vi "写入A1外设配置.vi"(8 "error in (no error)":errorcluster, 10 "外设配置":T1 {"总氮x公式0" items=["0", "1"]; "光谱仪类型" items=["1型", "2型", "3型", "2型氙灯联控"]; "泵阀量" items=["9通"=9, "10通"=10, "12通"=12]; "泵类型" items=["1型", "2型", "sy04型+旋转阀"]}, 11 "MB session in":refnum<class "MB_Master.lvclass">) -> (0 "error out":errorcluster, 3 "MB session out":refnum<class "MB_Master.lvclass">)   [LabVIEW 2016, in "斯坦道总磷总氮.lvlib"]
uses:
  <vilib>/Plasmionique/MB Master/MB_Master/MB_Master.lvclass
  <vilib>/Plasmionique/MB Master/MB_Master_Serial/MB_Master_Serial.lvclass
  C:/Program Files (x86)/National Instruments/LabVIEW 2016/vi.lib/Plasmionique/MB Master/MB_Master/MB_Master.lvclass
  <vilib>/Plasmionique/MB Master/MB Master.lvlib
  <vilib>/Utility/VariantDataType/VariantType.lvlib
panel:
  in  "U32":u32
  in  "SGL":sgl
  in  "U16":u16
  in  "U8":u8
  in  "VISA Resource":refnum<visa-resource-name>
  in  "引用选择":enum16{"MB引用", "自建引用"}(ring)
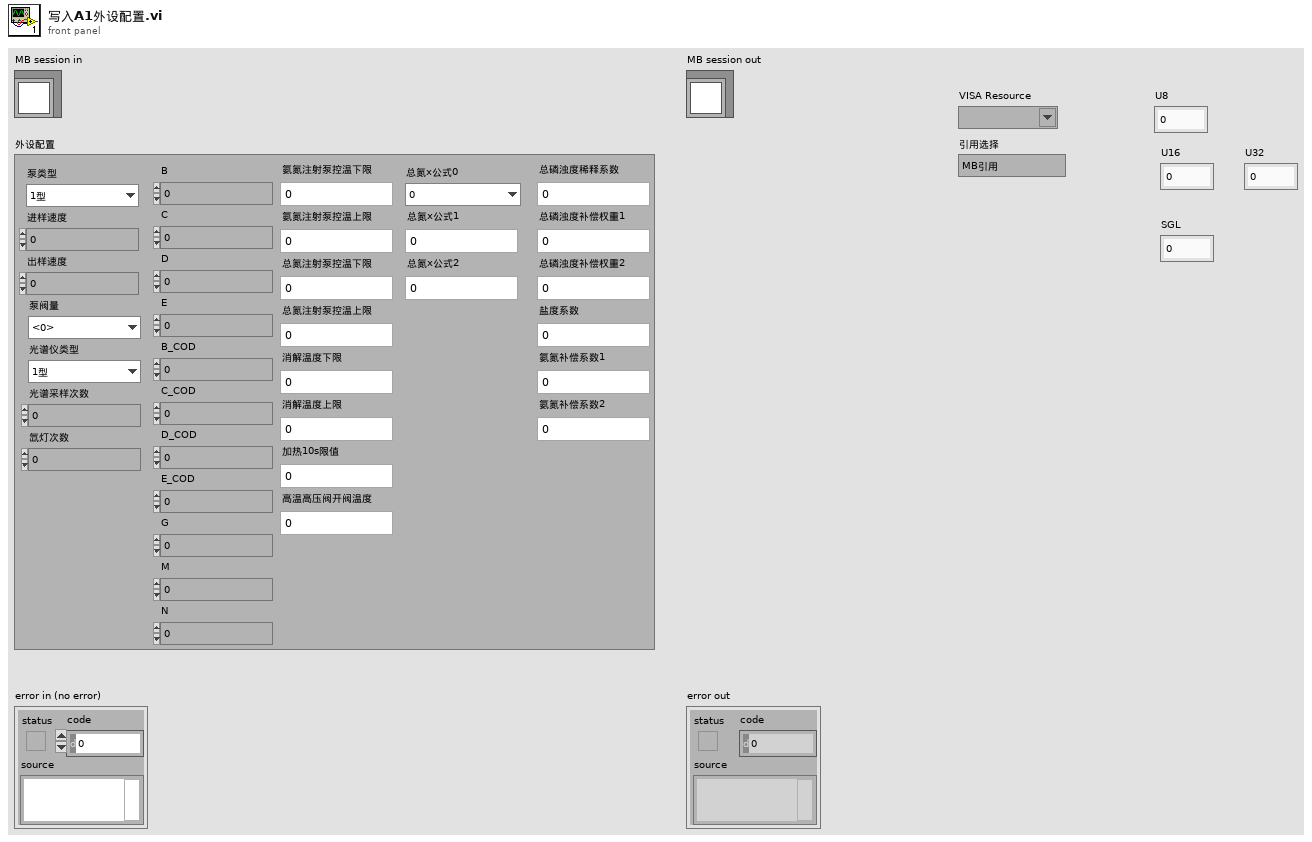
[diagram p1: front panel]
types:
  T1 = typedef "斯坦道总磷总氮.lvlib/V3 A1版外设参数.ctl" = cluster{"泵类型":u8, "进样速度":u32, "出样速度":u32, "泵阀量":u8, "光谱仪类型":u8, "光谱采样次数":u8, "氙灯次数":u8, "B":u16, "C":u16, "D":u16, "E":u16, "B_COD":u16, "C_COD":u16, "D_COD":u16, "E_COD":u16, "G":u16, "M":u16, "N":u16, "氨氮注射泵控温下限":sgl, "氨氮注射泵控温上限":sgl, "总氮注射泵控温下限":sgl, "总氮注射泵控温上限":sgl, "消解温度下限":sgl, "消解温度上限":sgl, "加热10s限值":sgl, "高温高压阀开阀温度":sgl, "总氮x公式0":u8, "总氮x公式1":sgl, "总氮x公式2":sgl, "总磷浊度稀释系数":sgl, "总磷浊度补偿权重1":sgl, "总磷浊度补偿权重2":sgl, "盐度系数":sgl, "氨氮补偿系数1":sgl, "氨氮补偿系数2":sgl}
  T2 = typedef "VariantType.lvlib/Type.ctl" = enum8{"Invalid Type", "Void", "I8", "I16", "I32", "I64", "U8", "U16", "U32", "U64", "Single Float", "Double Float", "Extended Float", "Single Complex", "Double Complex", "Extended Complex", "Enum U8", "Enum U16", "Enum U32", "Enum U64", "Single Float With Unit", "Double Float With Unit", "Extended Float With Unit", "Single Complex with Unit", "Double Complex with Unit", "Extended Complex with Unit", "Boolean", "String", "Path", "Picture", "Tag", "Array", "Cluster", "Variant", "LV Variant", "Waveform", "Timestamp", "Digital Waveform", "Digital Data", "ExpressData", "Refnum", "External Data", "VI", "Poly VI", "LabVIEW Class Instance", "Fixed Point"}
  T3 = cluster{"baud rate (bps)":u32, "stop bits":u16, "parity":u16, "flow control":u16, "timeout":u32, "retries":i32}
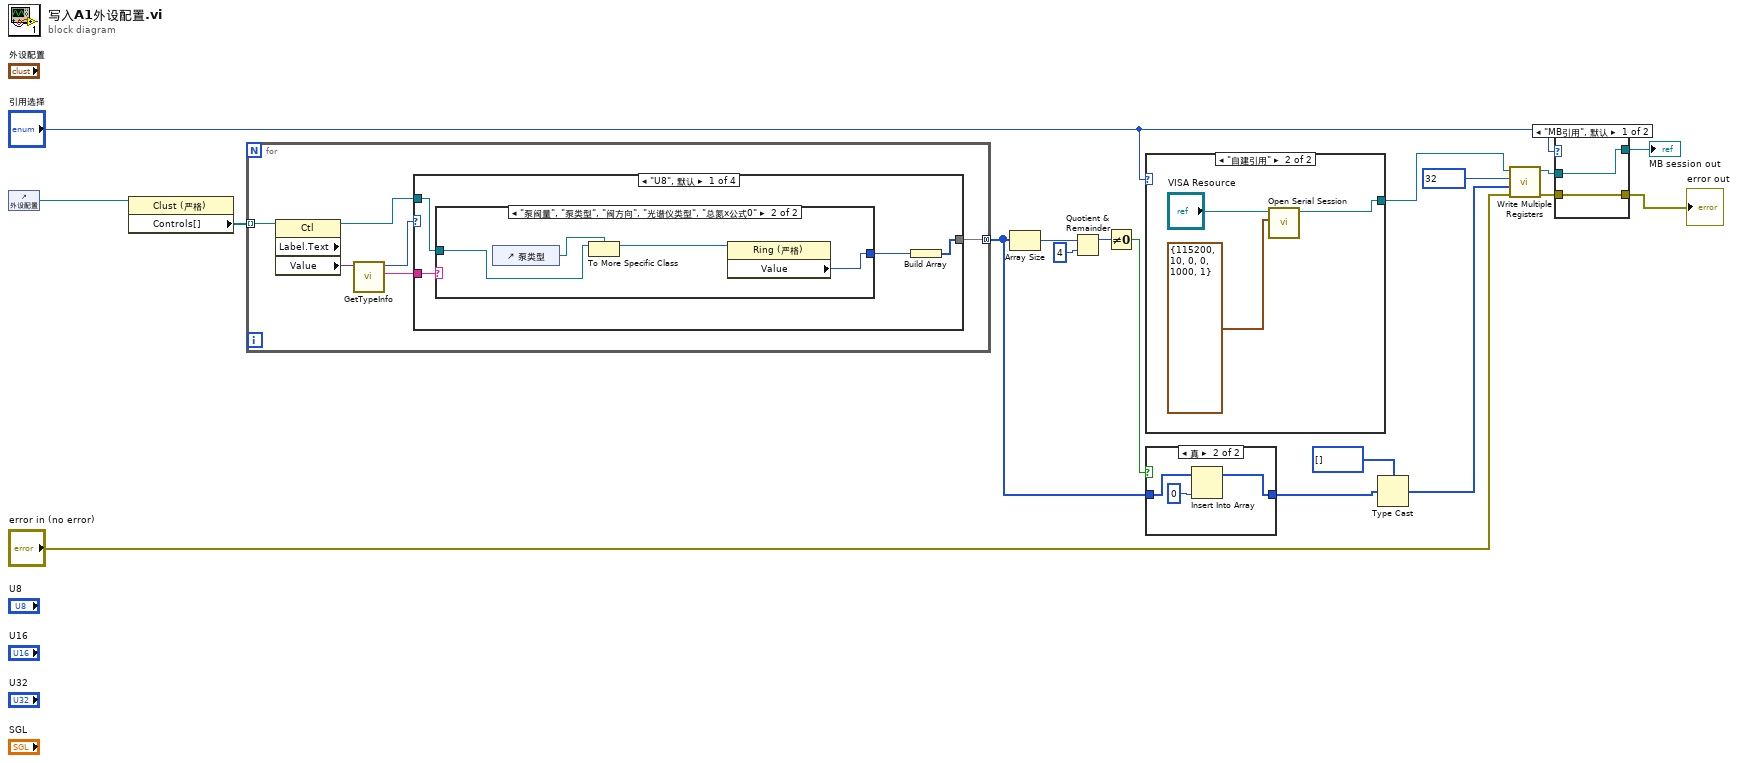
[diagram p0: block diagram]
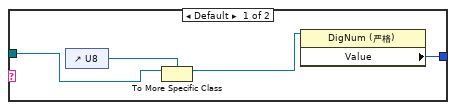
[diagram p3: hidden frame]
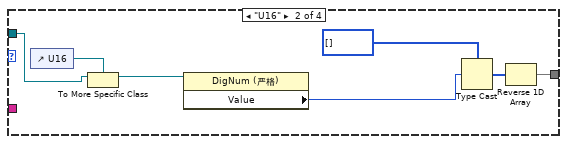
[diagram p4: hidden frame]
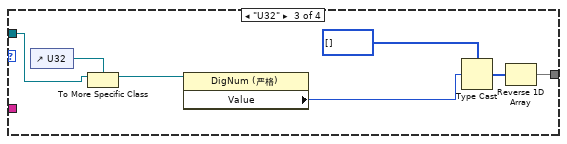
[diagram p5: hidden frame]
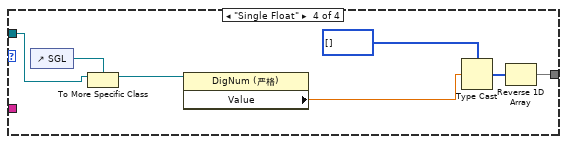
[diagram p6: hidden frame]
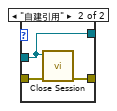
[diagram p7: hidden frame]
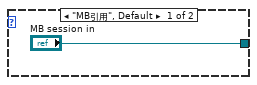
[diagram p8: hidden frame]
diagram:
  n1 = control-ref of="外设配置"() -> (w1:refnum<vi>)
  n2 = property class="Clust (严格)"(reference=w1) -> ("Controls[]"=w10:refnum<vi>[])  [unwired: 1 in, 2 out]
  n3 = for {
    tunnel: w10 -> [w24] mode=indexing
    tunnel: [w20] -> w3 mode=concatenating
    n4 = property class="Ctl" props=["Label", "Text", "Value"](reference=w24) -> (reference out=w21:refnum<vi>, "Value"=w23:variant)  [unwired: 1 in, 2 out]
    n5 = call <vilib>:"GetTypeInfo.vi"("Variant"=w23) -> ("Name"=w19:string, "Type Enum"=w22:T2)  [unwired: 6 in, 3 out]
    n6 = case shown="\"U8\", 默认" w22 {
      tunnel: w21 -> [w26 w43 w50 w57]
      tunnel: [w28 w37 w44 w51] -> w20
      tunnel: w19 -> [w27 _ _ _]
      frame "U8", Default {
        n7 = case shown="\"泵阀量\", \"泵类型\", \"阀方向\", \"光谱仪类型\", \"总氮x公式0\"" w27 {
          tunnel: w26 -> [w31 w36]
          tunnel: [w29 w33] -> w25
          frame Default {
            n8 = control-ref of="U8"() -> (w32:refnum<vi>)
            n9 = To More Specific Class(target class=w32, reference=w31) -> (specific class reference=w30:refnum<vi>)  [unwired: 1 in, 1 out]
            n10 = property class="DigNum (严格)"(reference=w30) -> ("Value"=w29:u8)  [unwired: 1 in, 2 out]
          }
          frame "泵阀量", "泵类型", "阀方向", "光谱仪类型", "总氮x公式0" {
            n11 = control-ref of="泵类型"() -> (w35:refnum<vi>)
            n12 = To More Specific Class(target class=w35, reference=w36) -> (specific class reference=w34:refnum<vi>)  [unwired: 1 in, 1 out]
            n13 = property class="Ring (严格)"(reference=w34) -> ("Value"=w33:u8)  [unwired: 1 in, 2 out]
          }
        }
        n14 = Build Array(w25) -> (w28:u8[])
      }
      frame "U16" {
        n15 = control-ref of="U16"() -> (w42:refnum<vi>)
        n16 = To More Specific Class(target class=w42, reference=w43) -> (specific class reference=w41:refnum<vi>)  [unwired: 1 in, 1 out]
        n17 = property class="DigNum (严格)"(reference=w41) -> ("Value"=w38:u16)  [unwired: 1 in, 2 out]
        n18 = Type Cast(type=u8[] [], x=w38) -> (*(type *) &x=w40:u8[])
        n19 = Reverse 1D Array(array=w40) -> (reversed array=w37:u8[])
      }
      frame "U32" {
        n20 = control-ref of="U32"() -> (w49:refnum<vi>)
        n21 = To More Specific Class(target class=w49, reference=w50) -> (specific class reference=w48:refnum<vi>)  [unwired: 1 in, 1 out]
        n22 = property class="DigNum (严格)"(reference=w48) -> ("Value"=w45:u32)  [unwired: 1 in, 2 out]
        n23 = Type Cast(type=u8[] [], x=w45) -> (*(type *) &x=w47:u8[])
        n24 = Reverse 1D Array(array=w47) -> (reversed array=w44:u8[])
      }
      frame "Single Float" {
        n25 = control-ref of="SGL"() -> (w56:refnum<vi>)
        n26 = To More Specific Class(target class=w56, reference=w57) -> (specific class reference=w55:refnum<vi>)  [unwired: 1 in, 1 out]
        n27 = property class="DigNum (严格)"(reference=w55) -> ("Value"=w52:sgl)  [unwired: 1 in, 2 out]
        n28 = Type Cast(type=u8[] [], x=w52) -> (*(type *) &x=w54:u8[])
        n29 = Reverse 1D Array(array=w54) -> (reversed array=w51:u8[])
      }
    }
  }
  n30 = Array Size(array=w3) -> (size(s)=w6:i32)
  n31 = Quotient & Remainder(x=w6, y=4) -> (x-y*floor(x/y)=w5:i32)  [unwired: 1 out]
  n32 = Not Equal To 0?(x=w5) -> (x != 0?=w4:bool)
  n33 = case shown="\"自建引用\"" "引用选择" {
    tunnel: ["MB session in" w61] -> w16
    frame "MB引用", Default {
    }
    frame "自建引用" {
      n34 = call <vilib>:"Open Serial Session.vi"("Serial Config"=T3 {"baud rate (bps)"=115200, "stop bits"=10, "parity"=0, "flow control"=0, "timeout"=1000, "retries"=1}, "VISA Resource"="VISA Resource") -> ("MB_Serial session"=w61:refnum<class "MB_Master_Serial.lvclass">)  [unwired: 8 in, 1 out]
    }
  }
  n35 = case shown="真" w4 {
    tunnel: w3 -> [w62 w65]
    tunnel: [w62 w63] -> w2
    frame False {
    }
    frame True {
      n36 = Insert Into Array(array=w65, new element=u8 0 ("新元素/子数组")) -> (w63:u8[])  [unwired: 1 in]
    }
  }
  n37 = Type Cast(type=u16[] [], x=w2) -> (*(type *) &x=w8:u16[])
  n38 = call <vilib>:"Write Multiple Registers.vi"("error in (no error)"="error in (no error)", "values"=w8, "starting address"=u16 32, "MB session in"=w16) -> ("error out"=w13:errorcluster, "MB session out"=w15:refnum<class "MB_Master.lvclass">)  [unwired: 6 in]
  n39 = case shown="\"MB引用\", 默认" "引用选择" {
    tunnel: w15 -> [w66 w68]
    tunnel: w13 -> [w67 w70]
    tunnel: [w67 w69] -> w12
    tunnel: [w66 w68] -> w11
    frame "MB引用", Default {
    }
    frame "自建引用" {
      n40 = call-dynamic "Close Session.vi"("error in (no error)"=w70, "MB session in"=w68) -> ("error out"=w69:errorcluster)  [unwired: 9 in]
    }
  }
  "MB session out" <- w11
  "error out" <- w12
